vi "NETWORK.vi"   [LabVIEW 2014]
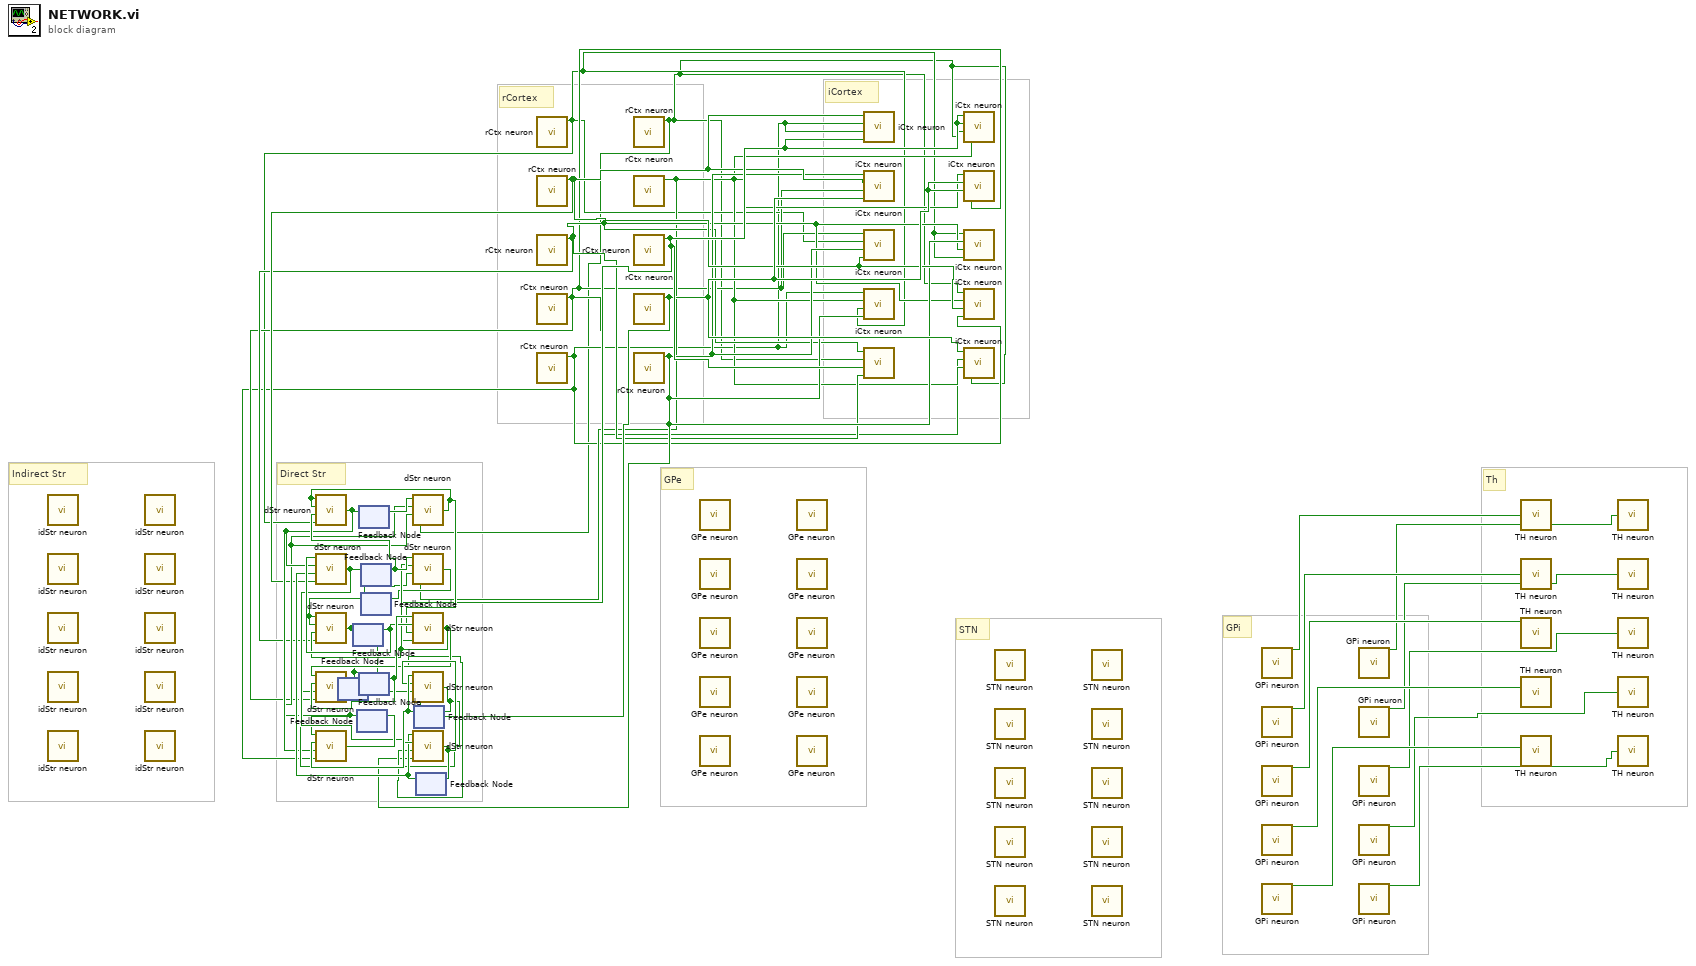
[diagram p0: block diagram]
diagram:
  # "STN"
  # "GPi"
  # "Direct Str"
  # "Indirect Str"
  # "GPe"
  # "rCortex"
  # "iCortex"
  # "Th"
  n1 = call "idStr neuron.vi"() -> ()  [unwired: 11 in, 1 out]
  n2 = call "idStr neuron.vi"() -> ()  [unwired: 11 in, 1 out]
  n3 = call "idStr neuron.vi"() -> ()  [unwired: 11 in, 1 out]
  n4 = call "idStr neuron.vi"() -> ()  [unwired: 11 in, 1 out]
  n5 = call "idStr neuron.vi"() -> ()  [unwired: 11 in, 1 out]
  n6 = call "idStr neuron.vi"() -> ()  [unwired: 11 in, 1 out]
  n7 = call "idStr neuron.vi"() -> ()  [unwired: 11 in, 1 out]
  n8 = call "idStr neuron.vi"() -> ()  [unwired: 11 in, 1 out]
  n9 = call "idStr neuron.vi"() -> ()  [unwired: 11 in, 1 out]
  n10 = call "idStr neuron.vi"() -> ()  [unwired: 11 in, 1 out]
  n11 = feedback #1() -> (w11:bool)  [unwired: 1 in]
  n12 = feedback #2() -> (w25:bool)  [unwired: 1 in]
  n13 = feedback #3() -> (w17:bool)  [unwired: 1 in]
  n14 = feedback #4() -> (w28:bool)  [unwired: 1 in]
  n15 = feedback-in #5(w11) -> ()
  n16 = feedback #5() -> (w27:bool)  [unwired: 1 in]
  n17 = feedback #6() -> (w22:bool)  [unwired: 1 in]
  n18 = feedback #7() -> (w15:bool)  [unwired: 1 in]
  n19 = feedback #8() -> (w26:bool)  [unwired: 1 in]
  n20 = feedback #9() -> (w21:bool)  [unwired: 1 in]
  n21 = call "rCtx neuron.vi"() -> ("Out"=w3:bool)  [unwired: 11 in]
  n22 = call "rCtx neuron.vi"() -> ("Out"=w8:bool)  [unwired: 11 in]
  n23 = call "rCtx neuron.vi"() -> ("Out"=w6:bool)  [unwired: 11 in]
  n24 = call "rCtx neuron.vi"() -> ("Out"=w4:bool)  [unwired: 11 in]
  n25 = call "rCtx neuron.vi"() -> ("Out"=w2:bool)  [unwired: 11 in]
  n26 = call "rCtx neuron.vi"() -> ("Out"=w1:bool)  [unwired: 11 in]
  n27 = call "dStr neuron.vi"("In 4"=w1, "In 3"=w17, "In 2"=w17, "In"=w28) -> ("Out"=w14:bool)
  n28 = call "dStr neuron.vi"("In 4"=w3, "In 3"=w22, "In 2"=w14, "In"=w14) -> ("Out"=w18:bool)
  n29 = call "dStr neuron.vi"("In 4"=w8, "In 3"=w21, "In 2"=w18, "In"=w25) -> ("Out"=w23:bool)
  n30 = call "dStr neuron.vi"("In 4"=w2, "In 3"=w18, "In 2"=w26, "In"=w17) -> ("Out"=w29:bool)
  n31 = feedback-in #3(w29) -> ()
  n32 = feedback-in #4(w18) -> ()
  n33 = feedback-in #6(w23) -> ()
  n34 = call "rCtx neuron.vi"() -> ("Out"=w5:bool)  [unwired: 11 in]
  n35 = call "rCtx neuron.vi"() -> ("Out"=w10:bool)  [unwired: 11 in]
  n36 = call "dStr neuron.vi"("In 4"=w10, "In 3"=w14, "In 2"=w25, "In"=w27) -> ("Out"=w20:bool)
  n37 = call "dStr neuron.vi"("In 4"=w6, "In 3"=w20, "In 2"=w15, "In"=w15) -> ("Out"=w13:bool)
  n38 = feedback-in #2(w13) -> ()
  n39 = call "dStr neuron.vi"("In 4"=w5, "In 3"=w15, "In 2"=w20, "In"=w22) -> ("Out"=w16:bool)
  n40 = feedback-in #7(w16) -> ()
  n41 = call "rCtx neuron.vi"() -> ("Out"=w9:bool)  [unwired: 11 in]
  n42 = call "rCtx neuron.vi"() -> ("Out"=w7:bool)  [unwired: 11 in]
  n43 = call "dStr neuron.vi"("In 4"=w7, "In 3"=w11, "In 2"=w23, "In"=w21) -> ("Out"=w24:bool)
  n44 = call "dStr neuron.vi"("In 4"=w9, "In 3"=w13, "In 2"=w24, "In"=w26) -> ("Out"=w19:bool)
  n45 = call "dStr neuron.vi"("In 4"=w4, "In 3"=w19, "In 2"=w27, "In"=w20) -> ("Out"=w12:bool)
  n46 = feedback-in #1(w12) -> ()
  n47 = feedback-in #8(w19) -> ()
  n48 = feedback-in #9(w24) -> ()
  n49 = call "GPe neuron.vi"() -> ()  [unwired: 27 in, 1 out]
  n50 = call "GPe neuron.vi"() -> ()  [unwired: 27 in, 1 out]
  n51 = call "GPe neuron.vi"() -> ()  [unwired: 27 in, 1 out]
  n52 = call "GPe neuron.vi"() -> ()  [unwired: 27 in, 1 out]
  n53 = call "GPe neuron.vi"() -> ()  [unwired: 27 in, 1 out]
  n54 = call "GPe neuron.vi"() -> ()  [unwired: 27 in, 1 out]
  n55 = call "GPe neuron.vi"() -> ()  [unwired: 27 in, 1 out]
  n56 = call "GPe neuron.vi"() -> ()  [unwired: 27 in, 1 out]
  n57 = call "GPe neuron.vi"() -> ()  [unwired: 27 in, 1 out]
  n58 = call "GPe neuron.vi"() -> ()  [unwired: 27 in, 1 out]
  n59 = call "iCtx neuron.vi"("In 4"=w10, "In 3"=w2, "In 2"=w2, "In"=w8) -> ()  [unwired: 1 out]
  n60 = call "iCtx neuron.vi"("In 4"=w9, "In 3"=w4, "In 2"=w8, "In"=w7) -> ()  [unwired: 1 out]
  n61 = call "iCtx neuron.vi"("In 4"=w8, "In 3"=w7, "In 2"=w3, "In"=w4) -> ()  [unwired: 1 out]
  n62 = call "iCtx neuron.vi"("In 4"=w7, "In 3"=w3, "In 2"=w5, "In"=w2) -> ()  [unwired: 1 out]
  n63 = call "iCtx neuron.vi"("In 4"=w6, "In 3"=w10, "In 2"=w1, "In"=w6) -> ()  [unwired: 1 out]
  n64 = call "iCtx neuron.vi"("In 4"=w5, "In 3"=w1, "In 2"=w10, "In"=w10) -> ()  [unwired: 1 out]
  n65 = call "iCtx neuron.vi"("In 4"=w4, "In 3"=w9, "In 2"=w9, "In"=w5) -> ()  [unwired: 1 out]
  n66 = call "iCtx neuron.vi"("In 4"=w3, "In 3"=w6, "In 2"=w7, "In"=w3) -> ()  [unwired: 1 out]
  n67 = call "iCtx neuron.vi"("In 4"=w2, "In 3"=w8, "In 2"=w6, "In"=w1) -> ()  [unwired: 1 out]
  n68 = call "iCtx neuron.vi"("In 4"=w1, "In 3"=w5, "In 2"=w4, "In"=w9) -> ()  [unwired: 1 out]
  n69 = call "STN neuron.vi"() -> ()  [unwired: 11 in, 1 out]
  n70 = call "STN neuron.vi"() -> ()  [unwired: 11 in, 1 out]
  n71 = call "STN neuron.vi"() -> ()  [unwired: 11 in, 1 out]
  n72 = call "STN neuron.vi"() -> ()  [unwired: 11 in, 1 out]
  n73 = call "STN neuron.vi"() -> ()  [unwired: 11 in, 1 out]
  n74 = call "STN neuron.vi"() -> ()  [unwired: 11 in, 1 out]
  n75 = call "STN neuron.vi"() -> ()  [unwired: 11 in, 1 out]
  n76 = call "STN neuron.vi"() -> ()  [unwired: 11 in, 1 out]
  n77 = call "STN neuron.vi"() -> ()  [unwired: 11 in, 1 out]
  n78 = call "STN neuron.vi"() -> ()  [unwired: 11 in, 1 out]
  n79 = call "GPi neuron.vi"() -> ("Out"=w39:bool)  [unwired: 27 in]
  n80 = call "GPi neuron.vi"() -> ("Out"=w38:bool)  [unwired: 27 in]
  n81 = call "GPi neuron.vi"() -> ("Out"=w37:bool)  [unwired: 27 in]
  n82 = call "GPi neuron.vi"() -> ("Out"=w36:bool)  [unwired: 27 in]
  n83 = call "GPi neuron.vi"() -> ("Out"=w35:bool)  [unwired: 27 in]
  n84 = call "GPi neuron.vi"() -> ("Out"=w34:bool)  [unwired: 27 in]
  n85 = call "GPi neuron.vi"() -> ("Out"=w33:bool)  [unwired: 27 in]
  n86 = call "GPi neuron.vi"() -> ("Out"=w32:bool)  [unwired: 27 in]
  n87 = call "GPi neuron.vi"() -> ("Out"=w31:bool)  [unwired: 27 in]
  n88 = call "GPi neuron.vi"() -> ("Out"=w30:bool)  [unwired: 27 in]
  n89 = call "TH neuron.vi"("In"=w39) -> ()  [unwired: 1 out]
  n90 = call "TH neuron.vi"("In"=w38) -> ()  [unwired: 1 out]
  n91 = call "TH neuron.vi"("In"=w37) -> ()  [unwired: 1 out]
  n92 = call "TH neuron.vi"("In"=w36) -> ()  [unwired: 1 out]
  n93 = call "TH neuron.vi"("In"=w35) -> ()  [unwired: 1 out]
  n94 = call "TH neuron.vi"("In"=w34) -> ()  [unwired: 1 out]
  n95 = call "TH neuron.vi"("In"=w33) -> ()  [unwired: 1 out]
  n96 = call "TH neuron.vi"("In"=w32) -> ()  [unwired: 1 out]
  n97 = call "TH neuron.vi"("In"=w31) -> ()  [unwired: 1 out]
  n98 = call "TH neuron.vi"("In"=w30) -> ()  [unwired: 1 out]
